vi "tables.vi"() -> ()   [LabVIEW 2014]
panel:
  in  "Final":dbl[](array[numeric])=[20.0, 40.0, 60.0]
  in  "Start":dbl[](array[numeric])=[0.001, 0.003, 0.005]
  in  "T":dbl[](array[numeric])=[50.0, 100.0, 150.0]
  in  "windows":dbl[](array[numeric])=[0.0, 0.15, 0.3]
  in  "Dcs":dbl[](array[numeric])=[0.0, 0.3, 0.6]
  out "Array":dbl[][](array[numeric])
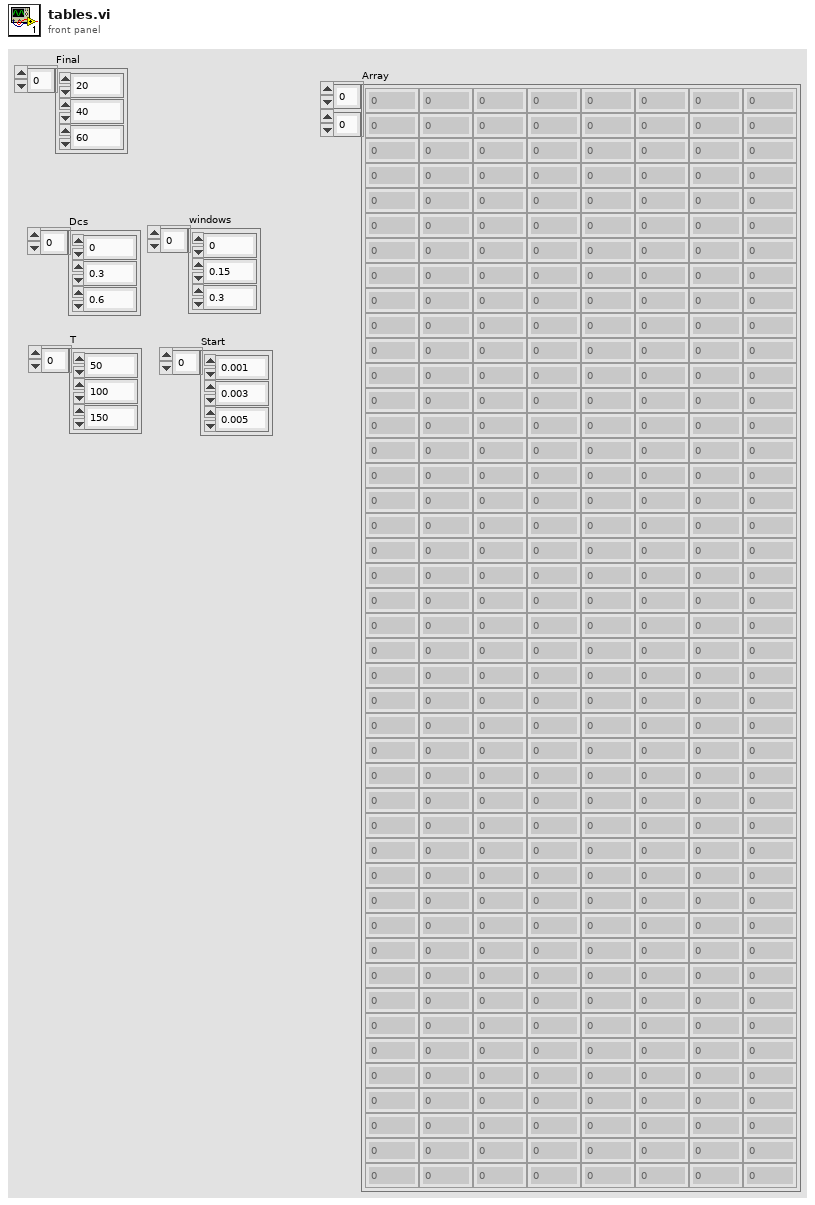
[diagram p1: front panel]
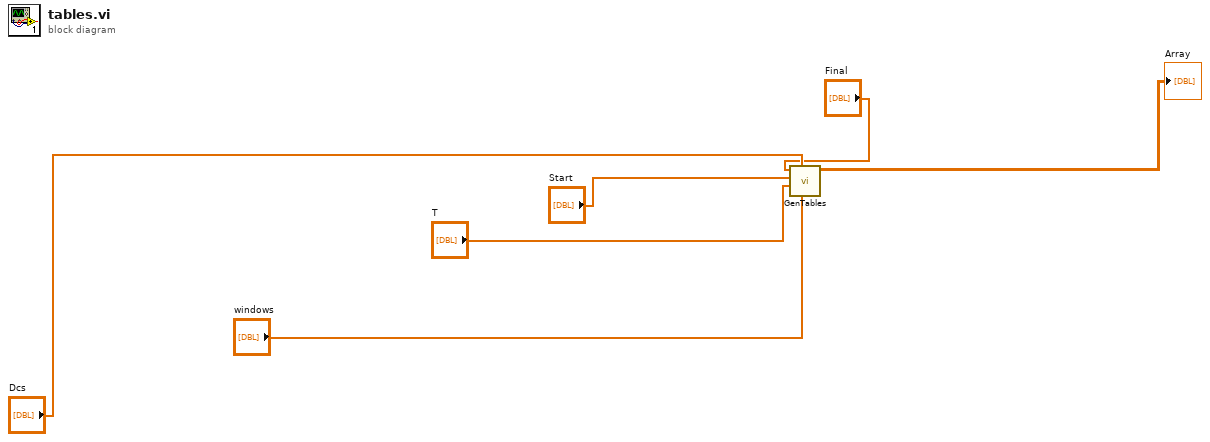
[diagram p0: block diagram]
diagram:
  n1 = call "GenTables.vi"("windows"="windows", "Dcs"="Dcs", "T"="T", "Start"="Start", "Final"="Final") -> ("Array"=→"Array":dbl[][])  [unwired: 6 in]
